vi "NumberOfGratingsGet.vi"(3 "error in (no error)":errorcluster, 5 "VISA resource name":refnum<visa-resource-name>) -> (0 "error out":errorcluster, 1 "Number of gratings":u8, 2 "VISA resource name out":refnum<visa-resource-name>)   [LabVIEW 2017, in "Spectral Products CM110.lvlib"]
uses:
  Spectral Products CM110.lvlib
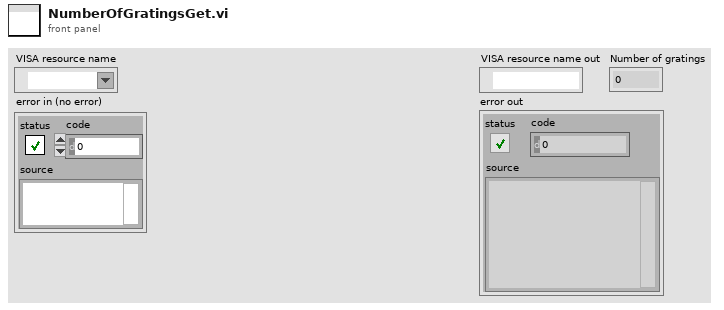
[diagram p1: front panel]
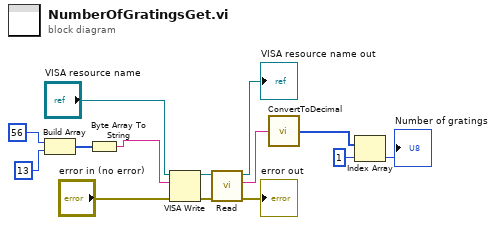
[diagram p0: block diagram]
diagram:
  n1 = Build Array(u8 56, u8 13) -> (w6:u8[])
  n2 = Byte Array To String(unsigned byte array=w6) -> (string=w4:string)
  n3 = VISA Write(VISA resource name="VISA resource name", write buffer=w4, error in (no error)="error in (no error)") -> (VISA resource name out=w13:refnum<visa-resource-name>, error out=w14:errorcluster)  [unwired: 1 out]
  n4 = call "Read.vi"("error in (no error)"=w14, "VISA Refnum in"=w13) -> ("error out"=→"error out":errorcluster, "read buffer"=w8:string, "VISA Refnum out"=→"VISA resource name out":refnum<visa-resource-name>)  [unwired: 6 in, 1 out]
  n5 = call "ConvertToDecimal.vi"("read buffer"=w8) -> ("unsigned byte array"=w3:u8[])
  n6 = Index Array(array=w3, index=1) -> (element=→"Number of gratings":u8)
